vi "去除无效数据.vi"   [LabVIEW 2018]
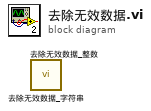
[diagram p0: block diagram]
diagram:
  n1 = call "去除无效数据_字符串.vi"() -> ()  [unwired: 11 in, 5 out]
  n2 = call "去除无效数据_整数.vi"() -> ()  [unwired: 11 in, 5 out]
